vi "TestExecuteTimedAvgSubscription_PublishOK.vi"(8 "error in (no error)":errorcluster, 11 "TestCase in":refnum<class "TestSubscriptionPolicy.lvclass">) -> (0 "error out":errorcluster, 3 "TestCase out":refnum<class "TestSubscriptionPolicy.lvclass">)   [LabVIEW 2015, in "SubscriptionPolicy.lvlib" / "TestSubscriptionPolicy.lvclass"]
uses:
  TestSubscriptionPolicy.lvclass
  TimedAverageSubscription/TimedAverageSubscription.lvclass/TimedAverageSubscription.ctl
  Components/TimedAverageBuffer/New Timed Average Buffer.vi
  TimedAverageSubscription/TimedAverageSubscription.lvclass
  Transport/QueueTransport/QueueTransport.lvclass
  IMediator/ISubscriptionPolicy/ISubscriptionPolicy.lvclass
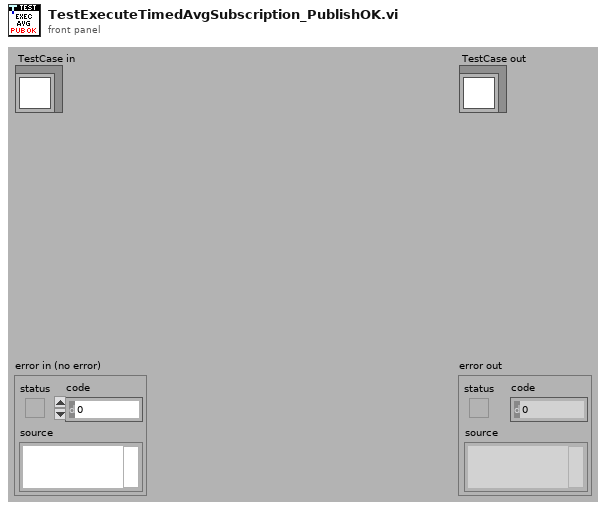
[diagram p1: front panel]
types:
  T1 = typedef "IMediator.lvlib/ISubscriptionPolicy.lvclass/ISubscriptionPolicy Reference.ctl" = refnum<data-value>
  T2 = cluster{"Data":variant, "Publication Time":timestamp}
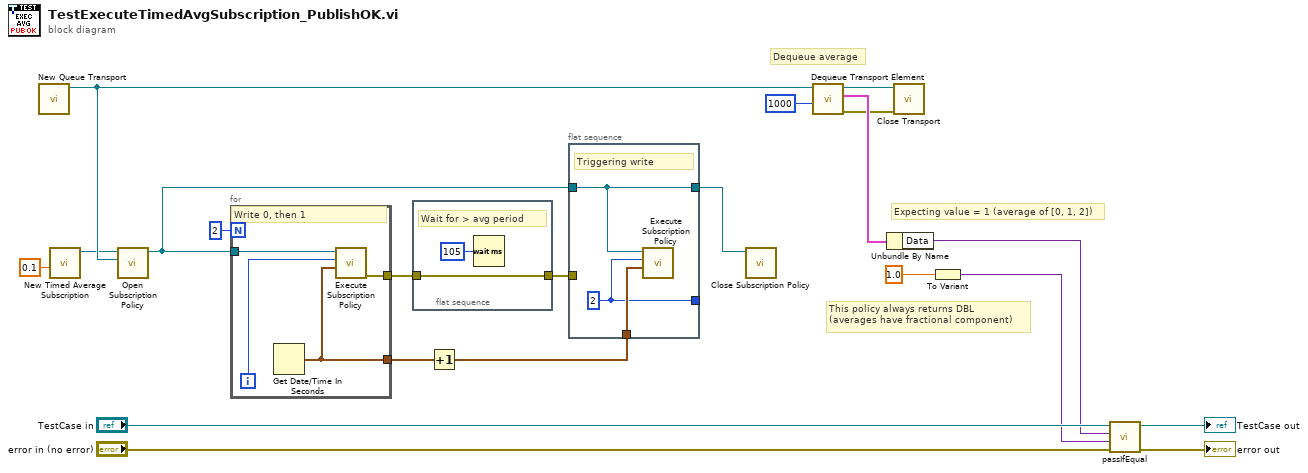
[diagram p0: block diagram]
diagram:
  # "This policy always returns DBL\n(averages have fractional component)"
  # "Dequeue average"
  # "Expecting value = 1 (average of [0, 1, 2])"
  n1 = call "New Queue Transport.vi"() -> ("QueueTransport Out"=w17:refnum<class "QueueTransport.lvclass">)  [unwired: 10 in, 1 out]
  n2 = call "New Timed Average Subscription.vi"("Average Period [s]"=0.1) -> ("TimedAverageSubscription Out"=w12:refnum<class "TimedAverageSubscription.lvclass">)  [unwired: 10 in]
  n3 = call "Open Subscription Policy.vi"("Transport"=w17, "SubscriptionPolicy"=w12) -> ("Subscription Policy"=w11:T1)  [unwired: 8 in, 1 out]
  n4 = for {
    N: 2 -> [_]
    tunnel: w11 -> [w25]
    tunnel: [w24] -> w10
    tunnel: [w23] -> w3
    i -> [w22]
    # "Write 0, then 1"
    n5 = Get Date/Time In Seconds() -> (seconds since 1Jan1904=w24:timestamp)
    n6 = call "Execute Subscription Policy.vi"("Publish Time"=w24, "New Topic Value"=w22, "Subscription Policy"=w25) -> ("error out (Unsubscribe?)"=w23:errorcluster)  [unwired: 8 in]
  }
  n7 = flat-sequence {
    tunnel: w3 -> [w27]
    tunnel: [w27] -> w2
    frame #0 {
      # "Wait for > avg period"
      n8 = Wait (ms)(milliseconds to wait=u32 105) -> ()  [unwired: 1 out]
    }
  }
  n9 = Increment(x=w10) -> (x+1=w9:timestamp)
  n10 = flat-sequence {
    tunnel: w11 -> [w28]
    tunnel: w9 -> [w30]
    tunnel: [w29] -> _
    tunnel: w2 -> [_]
    tunnel: [w28] -> w1
    frame #0 {
      w29 = 2
      # "Triggering write"
      n11 = call "Execute Subscription Policy.vi"("Publish Time"=w30, "New Topic Value"=w29, "Subscription Policy"=w28) -> ()  [unwired: 8 in, 1 out]
    }
  }
  n12 = call "Close Subscription Policy.vi"("Subscription Policy Reference"=w1) -> ()  [unwired: 10 in, 1 out]
  n13 = call "Dequeue Transport Element.vi"("Timeout In ms (-1)"=1000, "QueueTransport in"=w17) -> ("error out"=w13:errorcluster, "Element"=w15:T2, "QueueTransport out"=w14:refnum<class "QueueTransport.lvclass">)  [unwired: 6 in, 1 out]
  n14 = Unbundle By Name(w15) -> ("Data"=w6:variant)
  n15 = call-dynamic "Close Transport.vi"("error in (no error)"=w13, "QueueTransport in"=w14) -> ()  [unwired: 9 in, 1 out]
  n16 = To Variant(anything=1.0) -> (Variant=w4:variant)
  n17 = call-dynamic "passIfEqual.vi"("error in (no error)"="error in (no error)", "y"=w4, "x"=w6, "TestCase in"="TestCase in") -> ("error out"=→"error out":errorcluster, "TestCase out"=→"TestCase out":refnum<class "TestSubscriptionPolicy.lvclass">)  [unwired: 6 in]
